vi "_initializeLog.vi"(8 "error in (no error)":errorcluster, 11 "SkynetCompiler in":refnum<class "LVAutomationListener.lvclass">) -> (0 "error out":errorcluster, 3 "SkynetCompiler out":refnum<class "LVAutomationListener.lvclass">)   [LabVIEW 2013, in "LVAutomationListener.lvlib" / "LVAutomationListener.lvclass"]
uses:
  LVAutomationListener.lvclass
  LVAutomationListener.lvclass/LVAutomationListener.ctl
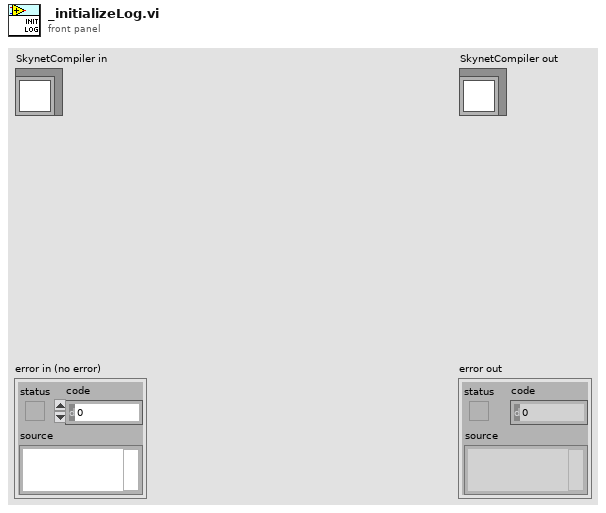
[diagram p1: front panel]
types:
  T1 = enum16{"open", "replace", "create", "open or create", "replace or create", "replace or create with confirmation"}
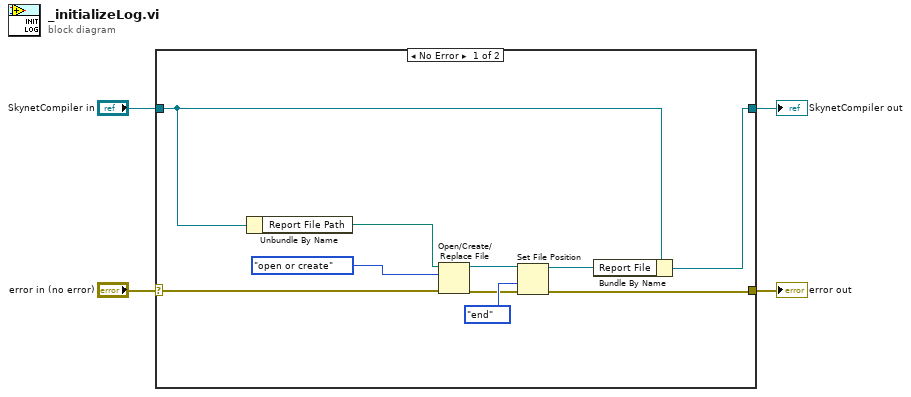
[diagram p0: block diagram]
diagram:
  n1 = case shown="No Error" "error in (no error)" {
    selector: "error in (no error)" -> [w10 w16]
    tunnel: [w9 w16] -> w3
    tunnel: [w6 w15] -> w1
    tunnel: "SkynetCompiler in" -> [w7 w15]
    frame No Error {
      n2 = Unbundle By Name(w7) -> ("Report File Path"=w8:path)
      n3 = Open/Create/Replace File(file path (use dialog)=w8, error in=w10, operation (0:open)=T1."open or create") -> (refnum out=w13:refnum<file>, error out=w12:errorcluster)  [unwired: 3 in, 1 out]
      n4 = Set File Position(refnum=w13, from (0:start)=enum16{"start", "end", "current"}."end", error in=w12) -> (refnum out=w5:refnum<file>, error out=w9:errorcluster)  [unwired: 1 in]
      n5 = Bundle By Name(cluster=w7, "Report File"=w5) -> (w6:refnum<class "LVAutomationListener.lvclass">)
    }
    frame Error {
    }
  }
  "error out" <- w3
  "SkynetCompiler out" <- w1
